vi "get_device_info.vi"(7 "info_options":T1, 9 "device_index":i32, 11 "error in (no error)":errorcluster) -> (8 "retrieved_info (str)":string, 15 "error out":errorcluster)   [LabVIEW 2012]
doc: "Retrieves device info based on device index. Device index is directly related to the order of all items found. \n\nImplementss the USB Communication API function \"fnPerformaxComGetProductString\".\n\nProduced By:\n\nChristopher Lemieux\nKod Integrations, LLC\n4835 Marianne Drive\nMount Airy, MD 21771\nhttp://www.kodintegrations.com\nemail: clemieux@kodintegrations.com\nphone: (240) 687-1288"
uses:
  support/controls/info_options.ctl
  support/controls/str_array_conv_actions.ctl
  support/controls/errors_actions.ctl
  PerformaxCom.dll
panel:
  in  "initialized_array":u8[](array[numeric])
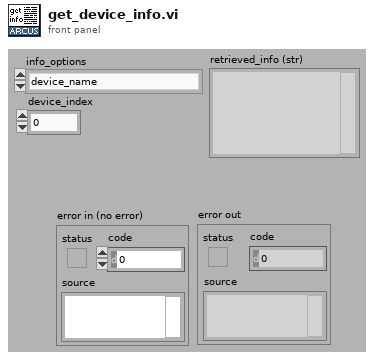
[diagram p1: front panel]
types:
  T1 = typedef "info_options.ctl" = enum16{"device_name", "description"}
  T2 = typedef "str_array_conv_actions.ctl" = enum16{"to_bytes", "to_string"}
  T3 = typedef "errors_actions.ctl" = enum16{"clearBuff", "closeRef", "noDeviceInfo", "noDevices", "openRef", "sendReceive", "setTimeouts", "unknown"}
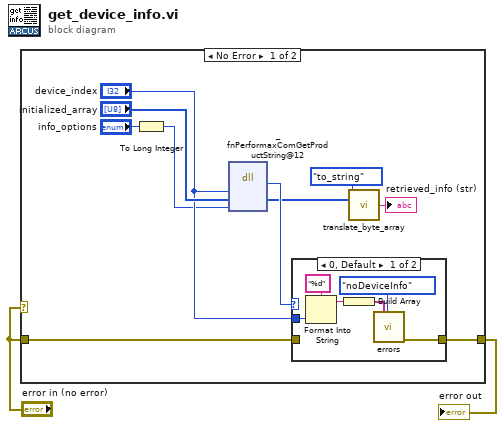
[diagram p0: block diagram]
diagram:
  n1 = case shown="No Error" "error in (no error)" {
    tunnel: "error in (no error)" -> [w10 w20]
    tunnel: [w9 w20] -> w1
    frame No Error {
      n2 = To Long Integer(number="info_options") -> (32bit integer=w6:i32)
      n3 = dll-call lib="PerformaxCom.dll" fn="_fnPerformaxComGetProductString@12"("devInd"="device_index", "returnedInfo"="initialized_array", "options"=w6) -> (w11:i32, "returnedInfo"=w5:u8[])  [unwired: 5 in, 2 out]
      n4 = case shown="0, Default" w11 {
        tunnel: [w17 w19] -> w9
        tunnel: w10 -> [_ w19]
        tunnel: "device_index" -> [w16 _]
        frame 0, Default {
          n5 = Format Into String(format string="%d", w16) -> (resulting string=w14:string)  [unwired: 2 in, 1 out]
          n6 = Build Array(w14) -> (w13:string[])
          n7 = call "errors.vi"("errors"=errors_actions."noDeviceInfo", "supp_text"=w13) -> ("error out"=w17:errorcluster)  [unwired: 13 in]
        }
        frame 1 {
        }
      }
      n8 = call "translate_byte_array.vi"("actions"=str_array_conv_actions."to_string", "byte_array (in)"=w5) -> ("string (out)"=→"retrieved_info (str)":string)  [unwired: 12 in, 1 out]
    }
    frame Error {
    }
  }
  "error out" <- w1
